vi "Video feed info class VI - retrieve video state.vi"(8 "error in (no error)":errorcluster, 11 "Video feed info in":refnum<class "Video feed info.lvclass">) -> (0 "error out":errorcluster, 2 "video state":T1(ring), 3 "Video feed info out":refnum<class "Video feed info.lvclass">)   [LabVIEW 2010, in "Video feed info.lvclass"]
uses:
  Video feed info.lvclass
  Video feed info.lvclass/Video feed info.ctl
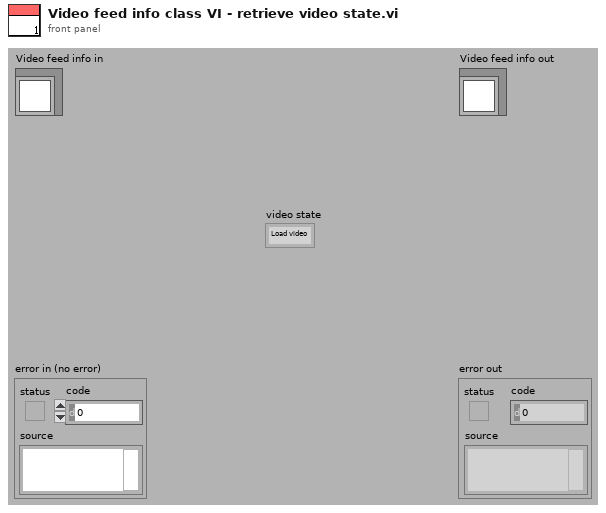
[diagram p1: front panel]
types:
  T1 = enum16{"Load video", "Idle", "Play", "Rewind", "Forward"}
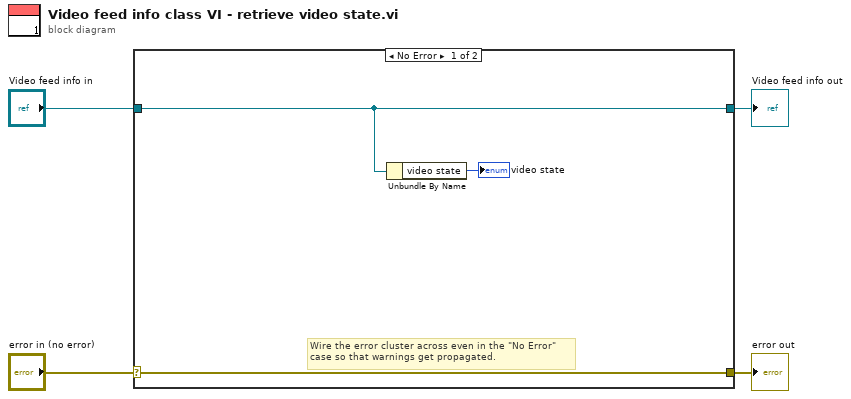
[diagram p0: block diagram]
diagram:
  n1 = case shown="No Error" "error in (no error)" {
    selector: "error in (no error)" -> [w7 w9]
    tunnel: [w7 w9] -> w3
    tunnel: [w6 w8] -> w1
    tunnel: "Video feed info in" -> [w6 w8]
    frame No Error {
      # "Wire the error cluster across even in the \"No Error\"\ncase so that warnings get propagated."
      n2 = Unbundle By Name(w6) -> ("video state"=→"video state":T1)
    }
    frame Error {
    }
  }
  "error out" <- w3
  "Video feed info out" <- w1
